vi "FormCmdPacket.vi"(5 "Cmd":string) -> (2 "Packet":string)   [LabVIEW 2018]
uses:
  Strict Type Controls/Settings Operation.ctl
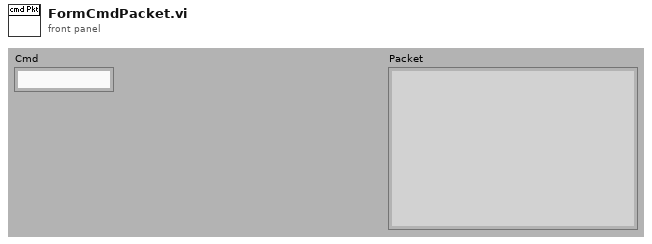
[diagram p1: front panel]
types:
  T1 = typedef "Settings Operation.ctl" = enum8{"Get Value", "Set Value", "Read File", "Write File", "Write Stored Value"}
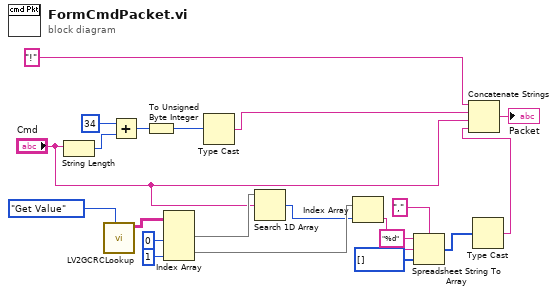
[diagram p0: block diagram]
diagram:
  n1 = String Length(string="Cmd") -> (length=w21:i32)
  n2 = call "LV2GCRCLookup.vi"("Operation"=Settings_Operation."Get Value") -> ("Lookup Out"=w17:string[][])  [unwired: 9 in, 1 out]
  n3 = Add(x=34, y=w21) -> (x+y=w19:i32)
  n4 = To Unsigned Byte Integer(number=w19) -> (unsigned 8bit integer=w10:u8)
  n5 = Index Array(array=w17, index (col) #1=0 ("disabled index (col)"), index (col) #2=1 ("index (col)")) -> (element #1=w14:string[], element #2=w13:string[])  [unwired: 2 in]
  n6 = Type Cast(x=w10) -> (*(type *) &x=w9:string)  [unwired: 1 in]
  n7 = Search 1D Array(1D array=w14, element="Cmd") -> (index of element=w12:i32)  [unwired: 1 in]
  n8 = Index Array(array=w13, index=w12) -> (element=w6:string)
  n9 = Spreadsheet String To Array(delimiter (Tab)=",", format string="%d", spreadsheet string=w6, array type (2D Dbl)=u8[] []) -> (array=w2:u8[])
  n10 = Type Cast(x=w2) -> (*(type *) &x=w1:string)  [unwired: 1 in]
  n11 = Concatenate Strings("!", w9, "Cmd", w1) -> (→"Packet":string)
